vi "Convert reley numbers to bool array.vi"(11 "Channels  numbers":u8[](array[numeric])) -> (2 "Channels converted":u8[](array[numeric]), 3 "Channels bool":bool[][](array[boolean]))   [LabVIEW 2020, in "DO_Relay.lvlib"]
uses:
  DO_Relay.lvlib
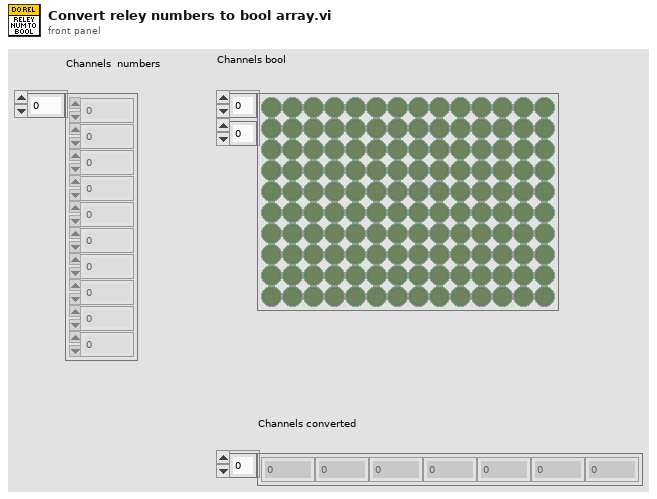
[diagram p1: front panel]
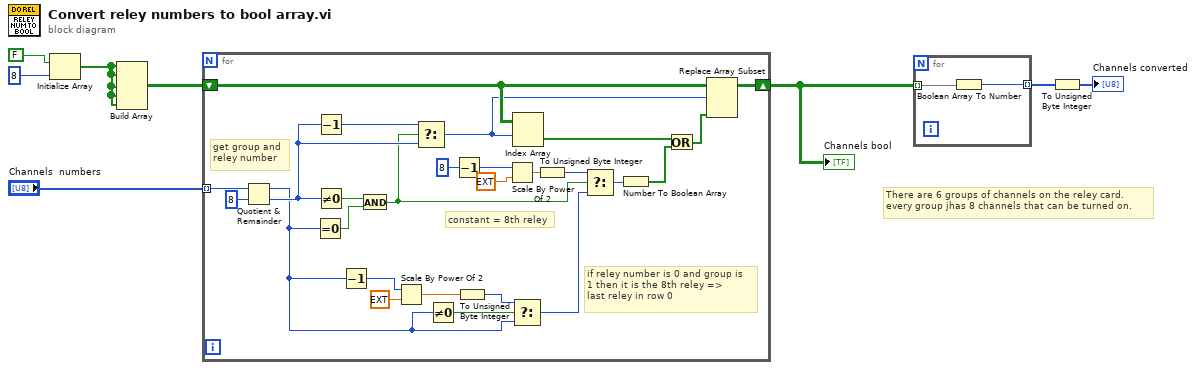
[diagram p0: block diagram]
diagram:
  # "There are 6 groups of channels on the reley card.\nevery group jhas 8 channels that can be turned on."
  n1 = Initialize Array(FALSE ("Boolean"), 8 ("dimension size")) -> (w5:bool[])
  n2 = Build Array(w5, w5, w5, w5, w5, w5) -> (w4:bool[][])
  n3 = for {
    tunnel: "Channels  numbers" -> [w21] mode=indexing
    shift-right: [w32] -> w3
    shift-left: w4 -> [w33]
    # "if reley number is 0 and group is\n1 then it is the 8th reley =>\nlast reley in row 0"
    # "get group and\nreley number"
    # "constant = 8th reley"
    n4 = Quotient & Remainder(x=w21, y=u8 8) -> (x-y*floor(x/y)=w18:u8, floor(x/y)=w27:u8)
    n5 = Equal To 0?(x=w18) -> (x = 0?=w10:bool)
    n6 = Decrement(x=w27) -> (x-1=w26:u8)
    n7 = Not Equal To 0?(x=w27) -> (x != 0?=w9:bool)
    n8 = Decrement(x=w18) -> (x-1=w22:u8)
    n9 = And(x=w9, y=w10) -> (x .and. y?=w11:bool)
    n10 = Scale By Power Of 2(n=w22, x=ext 1.0) -> (x*2^n=w20:ext)
    n11 = Select(t=w26, s=w11, f=w27) -> (s? t:f=w25:u8)
    n12 = Not Equal To 0?(x=w18) -> (x != 0?=w23:bool)
    n13 = Decrement(x=u8 8 ("t")) -> (x-1=w15:u8)
    n14 = To Unsigned Byte Integer(number=w20) -> (unsigned 8bit integer=w19:u8)
    n15 = Scale By Power Of 2(n=w15, x=ext 1.0) -> (x*2^n=w16:ext)
    n16 = Select(t=w19, s=w23, f=w18) -> (s? t:f=w17:u8)
    n17 = Index Array(array=w33, index (row)=w25) -> (element=w31:bool[])  [unwired: 1 in]
    n18 = To Unsigned Byte Integer(number=w16) -> (unsigned 8bit integer=w12:u8)
    n19 = Select(t=w12, s=w11, f=w17) -> (s? t:f=w24:u8)
    n20 = Number To Boolean Array(number=w24) -> (Boolean array=w30:bool[])
    n21 = Or(x=w31, y=w30) -> (x .or. y?=w29:bool[])
    n22 = Replace Array Subset(array=w33, new element=w29, index (row)=w25) -> (w32:bool[][])  [unwired: 1 in]
  }
  "Channels bool" <- w3
  n23 = for {
    tunnel: w3 -> [w36] mode=indexing
    tunnel: [w35] -> w2 mode=indexing
    n24 = Boolean Array To Number(Boolean array=w36) -> (number=w35:u32)
  }
  n25 = To Unsigned Byte Integer(number=w2) -> (unsigned 8bit integer=→"Channels converted":u8[])
